vi "Heater Power.vi"(8 "error in":errorcluster, 10 "On/Off":enum16{"Off", "On"}(ring), 11 "Neph in":refnum<class "Nephelometer.lvclass">) -> (0 "error out":errorcluster, 3 "Neph out":refnum<class "Nephelometer.lvclass">)   [LabVIEW 2014, in "Nephelometer.lvclass"]
uses:
  Nephelometer.lvclass
  Reusable/Session APIs/Serial/Serial Session.lvclass
  Nephelometer.lvclass/Nephelometer.ctl
  Accessors/Read Session Handle.vi
  <userlib>/_Session Fwk/Session - Root.lvclass
  Reusable/Session Log/System Log.lvclass
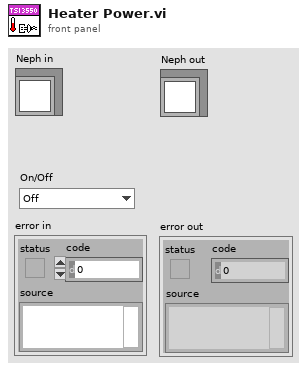
[diagram p1: front panel]
types:
  T1 = typedef "Session - Root.lvclass/Session Handle.ctl" = refnum<data-value>
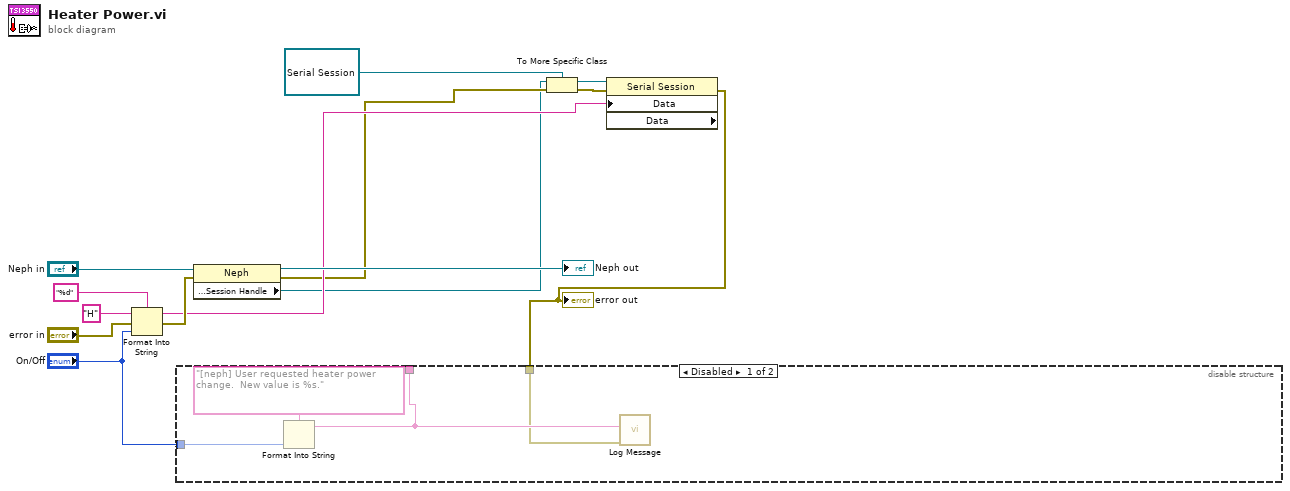
[diagram p0: block diagram]
diagram:
  n1 = Format Into String(format string="%d", initial string="H", error in="error in", "On/Off") -> (resulting string=w4:string, error out=w10:errorcluster)
  n2 = property class="Neph"(reference="Neph in", error in=w10) -> (reference out=→"Neph out":refnum<class "Nephelometer.lvclass">, error out=w3:errorcluster, "Accessors:Session Handle"=w2:T1)
  n3 = To More Specific Class(target class=refnum<data-value> refnum ("Session Handle"), reference=w2, error in=w3) -> (specific class reference=w6:refnum<data-value>, error out=w5:errorcluster)
  n4 = property class="Serial Session" props=["Data", "Data"](reference=w6, error in=w5, "Data"=w4) -> (error out=w1:errorcluster)  [unwired: 2 out]
  "error out" <- w1
  n5 = disable-structure shown="Disabled" {
    disable-tunnel: "On/Off" -> [w18 _]
    disable-tunnel: [w16 _] -> _
    disable-tunnel: w1 -> [w15 _]
    frame Disabled {
      n6 = Format Into String(format string="[neph] User requested heater power change.  New value is %s.", w18) -> (resulting string=w16:string)  [unwired: 2 in, 1 out]
      n7 = call "Log Message.vi"("error in"=w15, "MSG In"=w16) -> ()  [unwired: 8 in, 2 out]
    }
    frame Enabled {
    }
  }
